vi "DaqLink.vi"() -> ()   [LabVIEW 2009]
uses:
  Data Transmission/TransmissionState.ctl
  lib/Launcher/Launcher Actions.ctl
  lib/Launcher/NoPanelAppTypes.ctl
  lib/Data Access Objects/Metadata/Persistant DAO Actions.ctl
  lib/Apps/App Status Actions.ctl
panel:
  in  "Save":bool
  in  "Port Number":u16=6445
  out "Transmission State":T1=enum."Transmitting"
  out "Sending Data":bool
  in  "Wait For Notification Timeout":i32=1000000
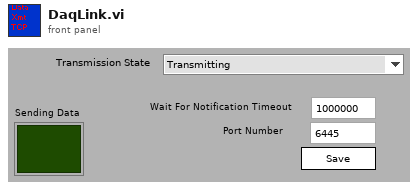
[diagram p1: front panel]
types:
  T1 = typedef "TransmissionState.ctl" = enum16{"Listening", "Transmitting", "Disconnecting"}
  T2 = typedef "Persistant DAO Actions.ctl" = enum16{"Init", "Get", "Set", "Load", "Save"}
  T3 = typedef "NoPanelAppTypes.ctl" = enum16{"NTCP Socket", "Data Archiving", "DAQ Link", "Control Loops", "Cmd Disp Diffs", "Individual Readings", "Limits"}
  T4 = typedef "Launcher Actions.ctl" = enum16{"Launch", "Stop All", "Stop", "Kill", "Running?", "Init"}
  T5 = typedef "Network Parameters.ctl" = cluster{"Port Number":u16, "Notification Name":string, "Wait For Notification Timeout":i32}
  T6 = typedef "App Status Actions.ctl" = enum16{"Init", "Get Status", "Running", "Control", "Autobalanced", "Data Acquisition", "Set App State", "DAQ Started", "Set LBCB State", "Set All", "Set Cont Logging", "Set Step Logging", "Set MM Logging", "Set Volt Logging", "Set Cart Type", "Set DAQ Link", "Set NTCP Link"}
  T7 = typedef "LBCB Location.ctl" = enum16{"Crane Bay Two LBCB", "Crane Bay One LBCB", "5th Scale Two LBCB", "5th Scale One LBCB", "Portable LBCB"}
  T8 = typedef "App Status.ctl" = cluster{"Running":bool, "Controlling L2":bool, "Autobalance L2":bool, "Data Acquisition":bool, " App State":T9, "DAQ Started":bool, "LBCB 1 State":T10, "LBCB 2 State":T10, "Controlling L1":bool, "Autobalance L1":bool, "Cartesian Type":bool, "Continuous Logging":bool, "Step Logging":bool, "Voltage Logging":bool, "Mixed Mode Logging":bool, "DAQ Link":bool, "NTCP Link ":bool}
  T9 = typedef "AppStates.ctl" = enum16{"Starting OM", "Initializing Displays", "Setting up Archiving", "Setting Up DAQ Channels", "Start DAQ", "DAQ Starting", "Controlling LBCBs", "Stopping OM"}
  T10 = typedef "Lbcb Control Loop States.ctl" = enum16{"Idle", "Start Selected", "Load Last Command", "Start Autobalancing", "Autobalancing", "Control Loop Initialized", "Control Enabled"}
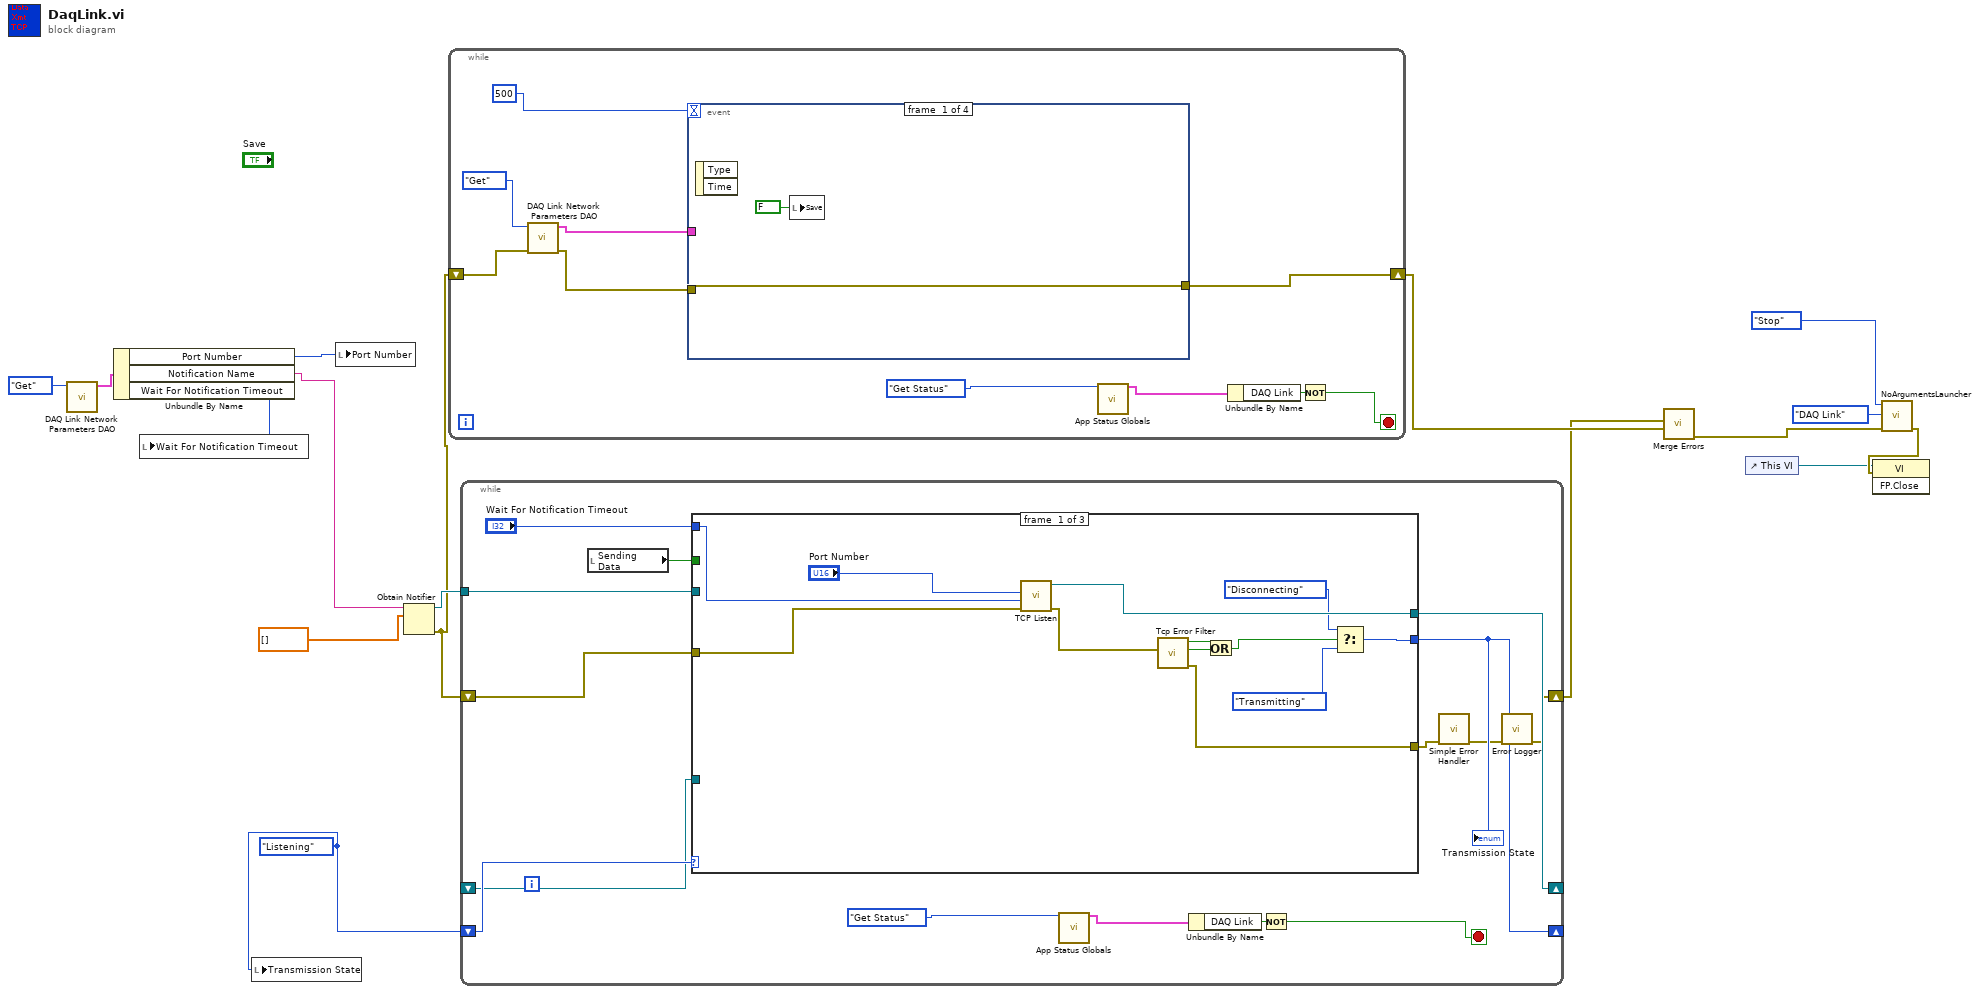
[diagram p0: block diagram]
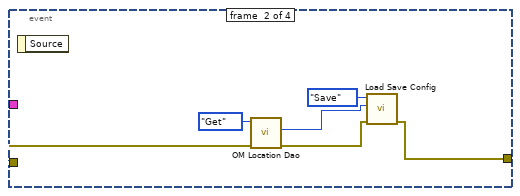
[diagram p2: hidden frame]
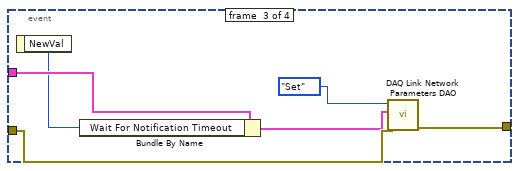
[diagram p3: hidden frame]
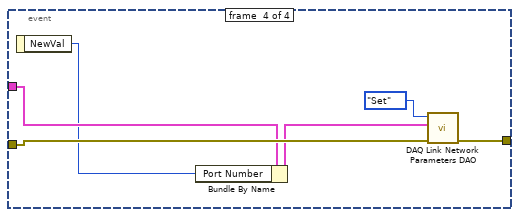
[diagram p4: hidden frame]
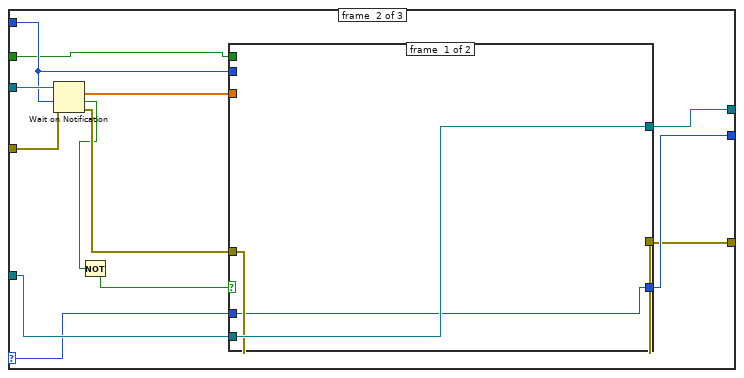
[diagram p5: hidden frame]
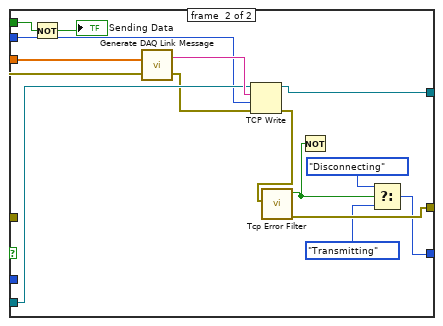
[diagram p6: hidden frame]
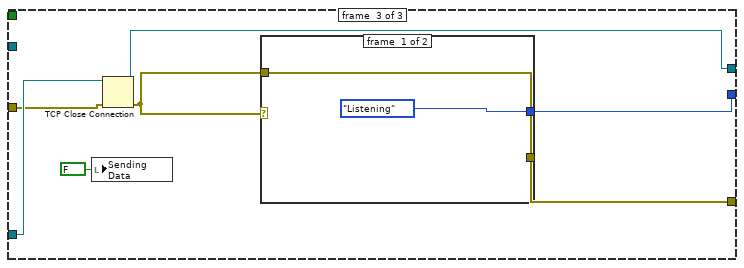
[diagram p7: hidden frame]
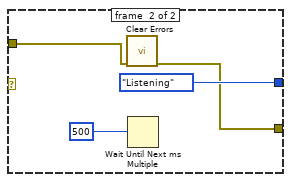
[diagram p8: hidden frame]
diagram:
  w15 = TransmissionState."Listening" ("Transmission State 2")
  n1 = call "DAQ Link Network Parameters DAO.vi"("Persistent DAO Actions"=Persistant_DAO_Actions."Get") -> ("Network Parameters Out"=w13:T5)  [unwired: 5 in, 5 out]
  n2 = Unbundle By Name(w13) -> ("Port Number"=w1:u16, "Notification Name"=w2:string, "Wait For Notification Timeout"=w3:i32)
  n3 = local write "Wait For Notification Timeout"(w3) -> ()
  n4 = local write "Transmission State"(w15) -> ()
  n5 = local write "Port Number"(w1) -> ()
  n6 = Obtain Notifier(name (unnamed)=w2, notification data type=dbl[] [] ("appended array")) -> (notifier out=w16:refnum<notifier>, error out=w5:errorcluster)  [unwired: 2 in, 1 out]
  n7 = while {
    shift-right: [w24] -> w8
    shift-left: w5 -> [w26]
    stop <- w19 stop-if-true
    n8 = call "DAQ Link Network Parameters DAO.vi"("error in (no error)"=w26, "Persistent DAO Actions"=Persistant_DAO_Actions."Get") -> ("error out"=w25:errorcluster, "Network Parameters Out"=w17:T5)  [unwired: 2 in, 6 out]
    n9 = event shown="[3] \"Port Number\": Value Change" {
      selector: _ -> [_ _ _ _]
      dyn-events: _ -> [_ _ _ _]
      timeout: 500 -> [_ _ _ _]
      tunnel: w25 -> [w28 w32 w40 w46]
      tunnel: [w28 w33 w39 w45] -> w24
      tunnel: w17 -> [_ _ w37 w43]
      event #0 {
        n10 = event-data() -> ()  [unwired: 3 out]
        n11 = local write "Save"(FALSE ("Save")) -> ()
      }
      event #1 {
        n12 = event-data() -> ()  [unwired: 2 out]
        n13 = call "OM Location Dao.vi"("error in (no error)"=w32, "Actions"=Persistant_DAO_Actions."Get") -> ("error out"=w31:errorcluster, "LBCB  Location Out"=w30:T7)  [unwired: 2 in, 6 out]
        n14 = call "Load Save Config.vi"("error in (no error)"=w31, "OM  Location"=w30, "Actions"=Persistant_DAO_Actions."Save") -> ("error out"=w33:errorcluster)  [unwired: 8 out]
      }
      event #2 {
        n15 = event-data() -> ("NewVal"=w35:i32)  [unwired: 1 out]
        n16 = Bundle By Name(cluster=w37, "Wait For Notification Timeout"=w35) -> (w36:T5)
        n17 = call "DAQ Link Network Parameters DAO.vi"("error in (no error)"=w40, "Network Parameters In"=w36, "Persistent DAO Actions"=Persistant_DAO_Actions."Set") -> ("error out"=w39:errorcluster)  [unwired: 2 in, 6 out]
      }
      event #3 {
        n18 = event-data() -> ("NewVal"=w41:u16)  [unwired: 1 out]
        n19 = Bundle By Name(cluster=w43, "Port Number"=w41) -> (w42:T5)
        n20 = call "DAQ Link Network Parameters DAO.vi"("error in (no error)"=w46, "Network Parameters In"=w42, "Persistent DAO Actions"=Persistant_DAO_Actions."Set") -> ("error out"=w45:errorcluster)  [unwired: 2 in, 6 out]
      }
    }
    n21 = call "App Status Globals.vi"("App Status Actions"=App_Status_Actions."Get Status") -> ("App Status Out"=w21:T8)  [unwired: 5 in, 9 out]
    n22 = Unbundle By Name(w21) -> ("DAQ Link"=w20:bool)
    n23 = Not(x=w20) -> (.not. x?=w19:bool)
  }
  n24 = while {
    shift-right: [w61] -> _
    shift-left: _ -> [w58]
    shift-right: [w53] -> w6
    shift-left: w5 -> [w60]
    shift-right: [w56] -> _
    shift-left: w15 -> [w59]
    tunnel: w16 -> [w57]
    stop <- w48 stop-if-true
    n25 = local read "Sending Data"() -> (w47:bool)
    n26 = case shown="\"Transmitting\"" w59 {
      selector: w59 -> [_ w76 _]
      tunnel: [w73 w82 w110] -> w61
      tunnel: w60 -> [w72 w85 w109]
      tunnel: [w63 w77 w106] -> w54
      tunnel: [w64 w78 w108] -> w56
      tunnel: w58 -> [_ w83 w111]
      tunnel: w57 -> [_ w86 _]
      tunnel: "Wait For Notification Timeout" -> [w71 w75 _]
      tunnel: w47 -> [_ w74 _]
      frame #0 {
        n27 = call <vilib>:"TCP Listen.vi"("error in (no error)"=w72, "timeout ms (wait forever: -1)"=w71, "port"="Port Number") -> ("error out"=w70:errorcluster, "connection ID"=w73:refnum<k5>)  [unwired: 1 in, 6 out]
        n28 = call "Tcp Error Filter.vi"("error in (no error)"=w70) -> ("error out"=w63:errorcluster, "Timed Out"=w68:bool, "Lost"=w69:bool)  [unwired: 8 out]
        n29 = Or(x=w69, y=w68) -> (x .or. y?=w67:bool)
        n30 = Select(t=TransmissionState."Disconnecting" ("Transmission State 2"), s=w67, f=TransmissionState."Transmitting" ("Transmission State 2")) -> (s? t:f=w64:T1)
      }
      frame #1 {
        n31 = Wait on Notification(notifier=w86, timeout in ms (-1)=w75, error in (no error)=w85) -> (notification=w84:dbl[], timed out?=w80:bool, error out=w81:errorcluster)  [unwired: 2 out]
        n32 = Not(x=w80) -> (.not. x?=w79:bool)
        n33 = case shown="True" w79 {
          tunnel: w84 -> [_ w100]
          tunnel: w83 -> [w89 w103]
          tunnel: [w89 w102] -> w82
          tunnel: w81 -> [w88 w101]
          tunnel: [w88 w96] -> w77
          tunnel: w75 -> [_ w98]
          tunnel: [w87 w92] -> w78
          tunnel: w76 -> [w87 _]
          tunnel: w74 -> [_ w90]
          frame #0 {
          }
          frame #1 {
            n34 = Not(x=w90) -> (.not. x?=→"Sending Data":bool)
            n35 = call "Generate DAQ Link Message.vi"("error in"=w101, "All Data"=w100) -> ("error out"=w99:errorcluster, "Message"=w104:string)
            n36 = TCP Write(connection ID=w103, data in=w104, error in (no error)=w99, 9:w98) -> (connection ID out=w102:refnum<k5>, error out=w97:errorcluster)  [unwired: 1 out]
            n37 = call "Tcp Error Filter.vi"("error in (no error)"=w97) -> ("error out"=w96:errorcluster, "Lost"=w94:bool)  [unwired: 9 out]
            n38 = Not(x=w94) -> ()  [unwired: 1 out]
            n39 = Select(t=TransmissionState."Disconnecting" ("Transmission State 2"), s=w94, f=TransmissionState."Transmitting" ("Transmission State 2")) -> (s? t:f=w92:T1)
          }
        }
      }
      frame #2 {
        n40 = local write "Sending Data"(FALSE ("Sending Data")) -> ()
        n41 = TCP Close Connection(connection ID=w111, error in (no error)=w109) -> (connection ID out=w110:refnum<k5>, error out=w107:errorcluster)  [unwired: 1 out]
        n42 = case shown="Error" w107 {
          tunnel: [TransmissionState."Listening" ("Transmission State 2") TransmissionState."Listening" ("Transmission State 2")] -> w108
          tunnel: w107 -> [w112 w115]
          tunnel: [w112 w114] -> w106
          frame #0 {
          }
          frame #1 {
            n43 = call <vilib>:"Clear Errors.vi"("error in (no error)"=w115) -> ("error out"=w114:errorcluster)  [unwired: 6 out]
            n44 = Wait Until Next ms Multiple(millisecond multiple=500) -> ()  [unwired: 1 out]
          }
        }
      }
    }
    "Transmission State" <- w56
    n45 = call "App Status Globals.vi"("App Status Actions"=App_Status_Actions."Get Status") -> ("App Status Out"=w50:T8)  [unwired: 5 in, 9 out]
    n46 = Unbundle By Name(w50) -> ("DAQ Link"=w49:bool)
    n47 = Not(x=w49) -> (.not. x?=w48:bool)
    n48 = call <vilib>:"Simple Error Handler.vi"("error in (no error)"=w54) -> ("error out"=w52:errorcluster)  [unwired: 1 in, 7 out]
    n49 = call "Error Logger.vi"("error in (no error)"=w52) -> ("error out"=w53:errorcluster)  [unwired: 1 in, 9 out]
  }
  n50 = call <vilib>:"Merge Errors.vi"("error in 3 (no error)"=w8, "error in 2 (no error)"=w6) -> ("error out"=w7:errorcluster)  [unwired: 2 in, 3 out]
  n51 = control-ref of="This VI"() -> (w11:refnum<vi>)
  n52 = call "NoArgumentsLauncher.vi"("error in (no error)"=w7, "Application"=NoPanelAppTypes."DAQ Link", "Application Launcher Actions"=Launcher_Actions."Stop") -> ("error out"=w12:errorcluster)  [unwired: 8 out]
  n53 = invoke class="VI" method="FP.Close"(reference=w11, error in=w12) -> ()  [unwired: 1 in, 3 out]
